vi "build_url_array.vi"(8 "error in (no error)":errorcluster, 11 "ComicVine_class in":refnum<class "series_class.lvclass">) -> (0 "error out":errorcluster, 2 "urls":string[](array[string]), 3 "ComicVine_class out":refnum<class "series_class.lvclass">)   [LabVIEW 2024, in "series_class.lvclass"]
uses:
  series_class.lvclass
  series_class.lvclass/series_class.ctl
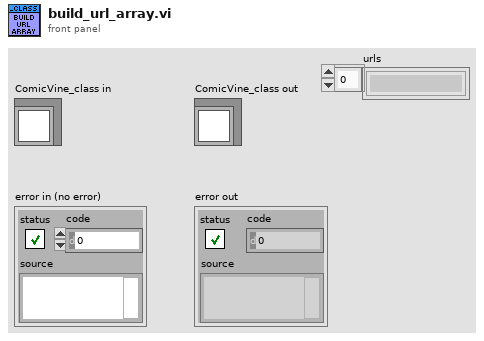
[diagram p1: front panel]
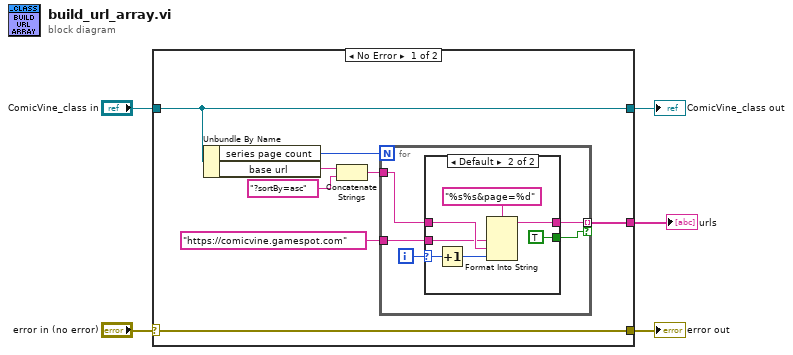
[diagram p0: block diagram]
diagram:
  n1 = case shown="No Error" "error in (no error)" {
    selector: "error in (no error)" -> [w13 w27]
    tunnel: [w13 w27] -> w4
    tunnel: [w6 w26] -> w2
    tunnel: "ComicVine_class in" -> [w6 w26]
    tunnel: [w7 _] -> w1
    frame No Error {
      n2 = Unbundle By Name(w6) -> ("series page count"=w12:i32, "base url"=w11:string)
      n3 = Concatenate Strings(w11, "?sortBy=asc") -> (w9:string)
      n4 = for {
        N: w12 -> [_]
        tunnel: w9 -> [w17]
        tunnel: [w16] -> w7 mode=indexing if=w14
        tunnel: "https://comicvine.gamespot.com" -> [w15]
        i -> [w18]
        n5 = case shown="Default" w18 {
          selector: w18 -> [_ w21]
          tunnel: w17 -> [_ w23]
          tunnel: [_ w24] -> w16
          tunnel: w15 -> [_ w22]
          tunnel: [_ TRUE] -> w14
          frame 0 {
          }
          frame Default {
            n6 = Increment(x=w21) -> (x+1=w20:i32)
            n7 = Format Into String(format string="%s%s&page=%d", w22, w23, w20) -> (resulting string=w24:string)  [unwired: 2 in, 1 out]
          }
        }
      }
    }
    frame Error {
    }
  }
  "error out" <- w4
  "ComicVine_class out" <- w2
  "urls" <- w1
